vi "GetAllUIStateChange.vi"(8 "error in (no error)":errorcluster, 11 "SMO.UI.MAUI in":refnum<class "SMO.UI.MAUI.lvclass">) -> (0 "error out":errorcluster, 2 "UIState":refnum<user-event>[](array[refnum]), 3 "SMO.UI.MAUI out":refnum<class "SMO.UI.MAUI.lvclass">)   [LabVIEW 2020, in "SMO.UI.MAUI.lvclass"]
uses:
  SMO.UI.MAUI.lvclass
  <vilib>/Levylab/SMO.UI.Embedded/SMO.UI.Embedded.lvclass
  <vilib>/Levylab/SMO.UI.Embedded/Typedefs/UI State.ctl
  <vilib>/Levylab/SMO.UI.Embedded/Typedefs/PublicEvents--SMO.UI.Embedded.UIState.ctl
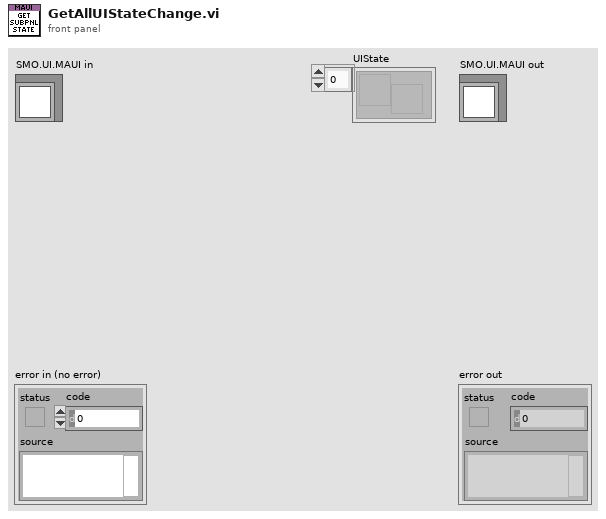
[diagram p1: front panel]
types:
  T1 = typedef "SMO.UI.Embedded.lvclass/PublicEvents--Cluster.ctl" = cluster{"ReadyForInfo":refnum<user-event>, "UIState":refnum<user-event>}
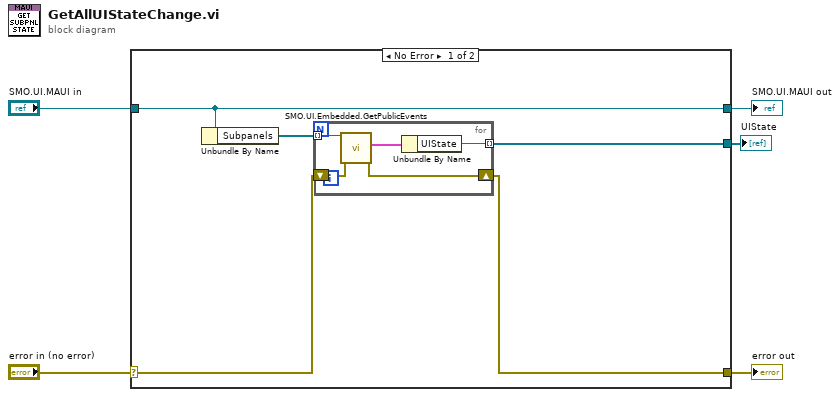
[diagram p0: block diagram]
diagram:
  n1 = case shown="No Error" "error in (no error)" {
    selector: "error in (no error)" -> [w7 w17]
    tunnel: [w6 w17] -> w4
    tunnel: [w10 w16] -> w2
    tunnel: "SMO.UI.MAUI in" -> [w10 w16]
    tunnel: [w8 _] -> w1
    frame No Error {
      n2 = Unbundle By Name(w10) -> ("Subpanels"=w9:refnum<class "SMO.UI.Embedded.lvclass">[])
      n3 = for {
        tunnel: w9 -> [w15] mode=indexing
        tunnel: [w13] -> w8 mode=indexing
        shift-right: [w11] -> w6
        shift-left: w7 -> [w12]
        n4 = call <vilib>:"SMO.UI.Embedded.GetPublicEvents.vi"("error in (no error)"=w12, "EmbeddedSMO"=w15) -> ("error out"=w11:errorcluster, "Public Events"=w14:T1)  [unwired: 7 in, 1 out]
        n5 = Unbundle By Name(w14) -> ("UIState"=w13:refnum<user-event>)
      }
    }
    frame Error {
    }
  }
  "error out" <- w4
  "SMO.UI.MAUI out" <- w2
  "UIState" <- w1
